vi "power_measure.vi"() -> ()   [LabVIEW 2020]
uses:
  <vilib>/ptbypt/NI_PtbyPt.lvlib
panel:
  in  "save":bool
  in  "no of data point for time":i32=100
  in  "no. of  data point for power":i32=100
  out "Avg_time":dbl format="%0.2f"
  out "average_power":dbl
  out "Time (s)":dbl
  out "Date":string
  in  "Filename":string
  in  "path":path
  out "Waveform Chart":waveform(dbl)(graph)
  out "Power":dbl
  in  "stop":bool
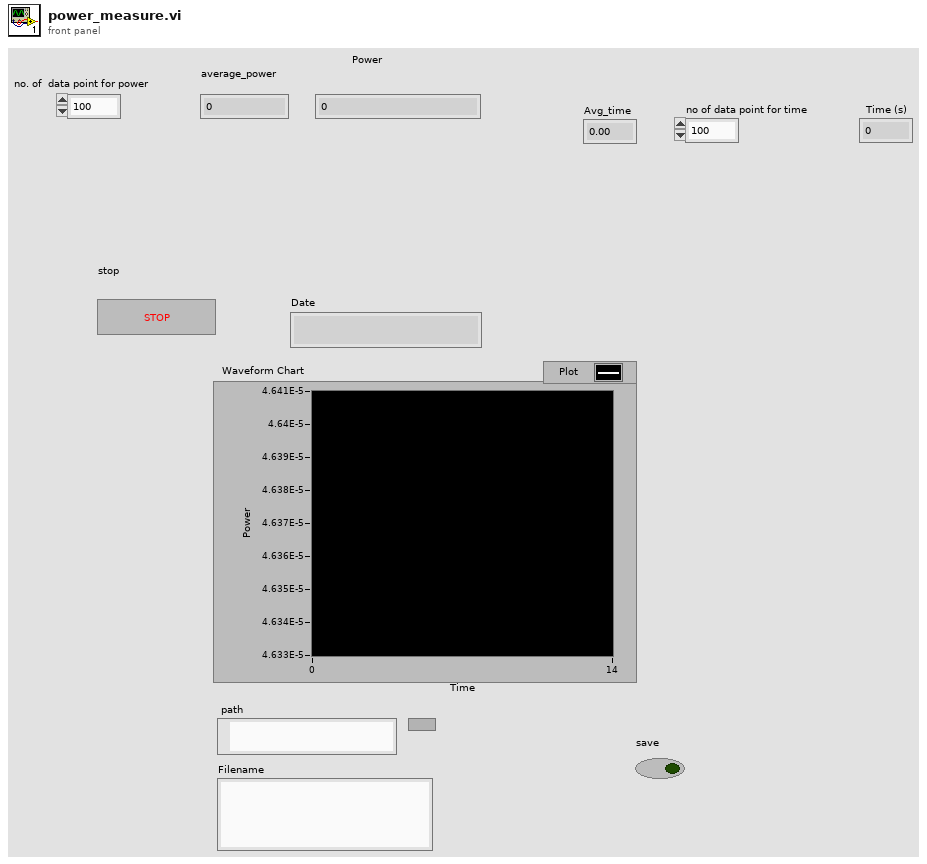
[diagram p1: front panel]
types:
  T1 = enum16{"open", "replace", "create", "open or create", "replace or create", "replace or create with confirmation"}
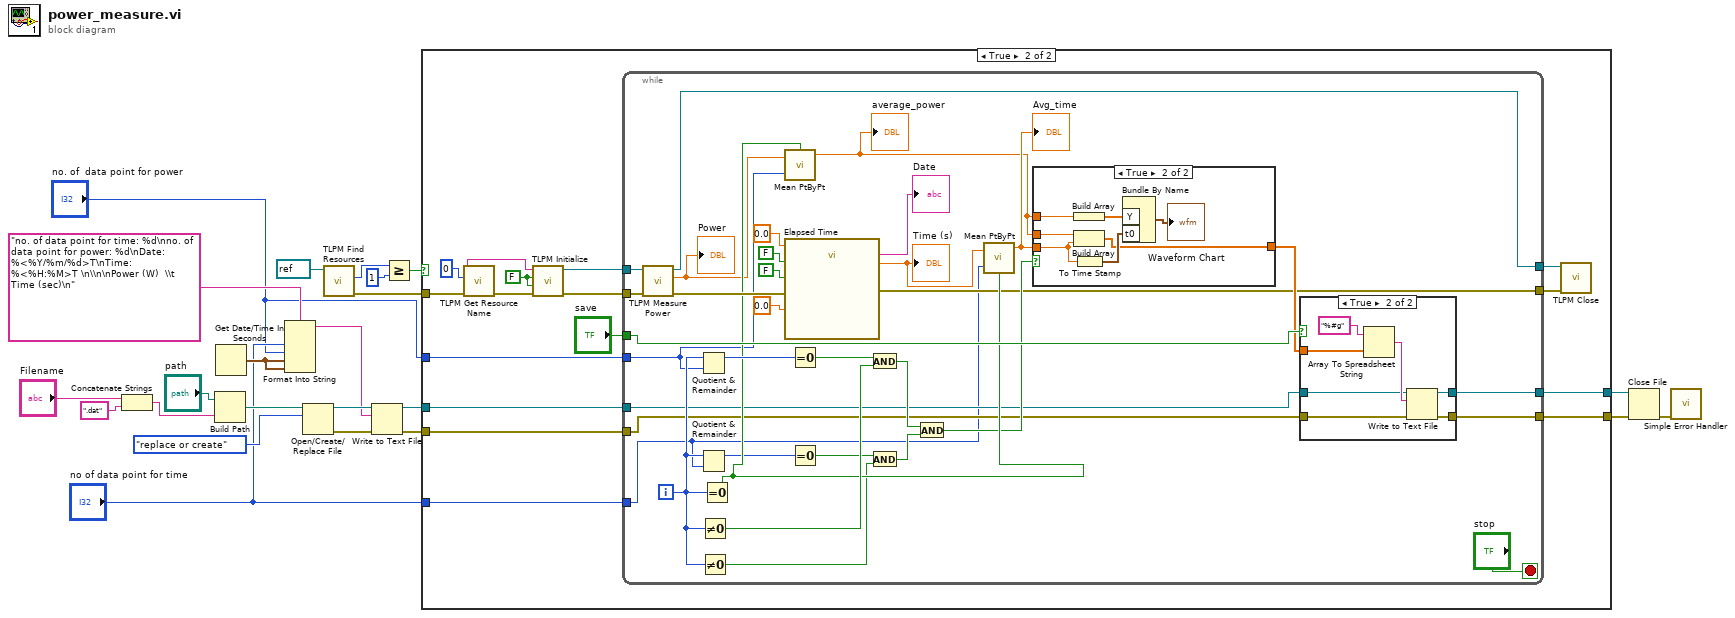
[diagram p0: block diagram]
diagram:
  n1 = Concatenate Strings("Filename", ".dat" ("string")) -> (w17:string)
  n2 = Build Path(base path="path", name or relative path=w17) -> (appended path=w14:path)
  n3 = Get Date/Time In Seconds() -> (seconds since 1Jan1904=w5:timestamp)
  n4 = Format Into String(format string="no. of data point for time: %d\nno. of data point for power: %d\nDate: %<%Y/%m/%d>T\nTime: %<%H:%M>T \n\\n\nPower (W)  \\t  Time (sec)\n", "no of data point for time", "no. of  data point for power", w5, w5) -> (resulting string=w3:string)  [unwired: 2 in, 1 out]
  n5 = Open/Create/Replace File(file path (use dialog)=w14, operation (0:open)=T1."replace or create") -> (refnum out=w12:refnum<file>, error out=w11:errorcluster)  [unwired: 4 in, 1 out]
  n6 = call <instrlib>:"TLPM Find Resources.vi"("instrument handle"=refnum<visa-resource-name> refnum) -> ("error out"=w15:errorcluster, "Resource Count"=w21:u32)  [unwired: 8 in, 1 out]
  n7 = Write to Text File(file (use dialog)=w12, text=w3, error in=w11) -> (refnum out=w10:refnum<file>, error out=w8:errorcluster)  [unwired: 1 in, 1 out]
  n8 = Greater Or Equal?(x=w21, y=u32 1) -> (x >= y?=w22:bool)
  n9 = case shown="True" w22 {
    tunnel: w15 -> [_ w34]
    tunnel: w10 -> [w24 w32]
    tunnel: [w24 w31] -> w9
    tunnel: w8 -> [w25 w30]
    tunnel: [w25 w29] -> w7
    tunnel: "no. of  data point for power" -> [_ w28]
    tunnel: "no of data point for time" -> [_ w27]
    frame False {
    }
    frame True {
      w37 = FALSE ("ID Query (Do Query)")
      n10 = call <instrlib>:"TLPM Get Resource Name.vi"("error in (no error)"=w34, "Index (0)"=u32 0) -> ("error out"=w35:errorcluster, "Resource Name"=w40:string)  [unwired: 7 in, 1 out]
      n11 = call <instrlib>:"TLPM Initialize.vi"("error in (no error)"=w35, "Reset Device (Reset Device)"=w37, "ID Query (Do Query)"=w37, "resource name"=w40) -> ("error out"=w36:errorcluster, "instrument handle out"=w39:refnum<visa-resource-name>)  [unwired: 6 in]
      n12 = while {
        tunnel: w39 -> [w74]
        tunnel: [w73] -> w38
        tunnel: "save" -> [w71]
        tunnel: w36 -> [w72]
        tunnel: [w50] -> w33
        tunnel: w32 -> [w49]
        tunnel: [w48] -> w31
        tunnel: w30 -> [w47]
        tunnel: [w46] -> w29
        tunnel: w28 -> [w45]
        tunnel: w27 -> [w42]
        i -> [w58]
        stop <- "stop" stop-if-true
        n13 = call <instrlib>:"TLPM Measure Power.vi"("error in (no error)"=w72, "instrument handle"=w74) -> ("error out"=w70:errorcluster, "Power"=w44:dbl, "instrument handle out"=w73:refnum<visa-resource-name>)  [unwired: 7 in]
        "Power" <- w44
        n14 = Quotient & Remainder(x=w58, y=w45) -> (x-y*floor(x/y)=w64:i32)  [unwired: 1 out]
        n15 = Quotient & Remainder(x=w58, y=w42) -> (x-y*floor(x/y)=w59:i32)  [unwired: 1 out]
        n16 = Not Equal To 0?(x=w58) -> (x != 0?=w62:bool)
        n17 = Not Equal To 0?(x=w58) -> (x != 0?=w56:bool)
        n18 = Equal To 0?(x=w58) -> (x = 0?=w61:bool)
        n19 = call <vilib>:"Mean PtByPt.vi"("x"=w44, "sample length"=w45, "initialize"=w61) -> ("mean"=w52:dbl)  [unwired: 1 in, 1 out]
        "average_power" <- w52
        n20 = call "Elapsed Time"("Time Target (s)"=0.0, "Reset"=FALSE ("Auto Reset"), "Auto Reset"=FALSE ("Reset"), "error in (no error)"=w70, "Set Start Time (s)"=0.0) -> ("Present Text"=→"Date":string, "Elapsed Time (s)"=w43:dbl, "error out"=w50:errorcluster)  [unwired: 7 in, 5 out]
        "Time (s)" <- w43
        n21 = Equal To 0?(x=w64) -> (x = 0?=w63:bool)
        n22 = Equal To 0?(x=w59) -> (x = 0?=w57:bool)
        n23 = And(x=w63, y=w62) -> (x .and. y?=w54:bool)
        n24 = And(x=w57, y=w56) -> (x .and. y?=w55:bool)
        n25 = And(x=w54, y=w55) -> (x .and. y?=w53:bool)
        n26 = call <vilib>:"Mean PtByPt.vi"("x"=w43, "sample length"=w42, "initialize"=w61) -> ("mean"=w60:dbl)  [unwired: 1 in, 1 out]
        "Avg_time" <- w60
        n27 = case shown="True" w53 {
          tunnel: w52 -> [_ w81]
          tunnel: w60 -> [_ w78]
          tunnel: w52 -> [_ w77]
          tunnel: [_ w76] -> w51
          frame False {
          }
          frame True {
            n28 = Build Array(w81) -> (w80:dbl[])
            n29 = Build Array(w77, w78) -> (w76:dbl[])
            n30 = To Time Stamp(1:w78) -> (0:w79:timestamp)
            n31 = Bundle By Name("Y"=w80, "t0"=w79) -> (→"Waveform Chart":waveform(dbl))  [unwired: 1 in]
          }
        }
        n32 = case shown="True" w71 {
          tunnel: w51 -> [_ w89]
          tunnel: w49 -> [w83 w88]
          tunnel: [w83 w87] -> w48
          tunnel: w47 -> [w84 w86]
          tunnel: [w84 w85] -> w46
          frame False {
          }
          frame True {
            n33 = Array To Spreadsheet String(array=w89, 3:"%#g" ("format string")) -> (spreadsheet string=w91:string)  [unwired: 1 in]
            n34 = Write to Text File(file (use dialog)=w88, text=w91, error in=w86) -> (refnum out=w87:refnum<file>, error out=w85:errorcluster)  [unwired: 1 in, 1 out]
          }
        }
      }
      n35 = call <instrlib>:"TLPM Close.vi"("error in (no error)"=w33, "instrument handle"=w38) -> ()  [unwired: 9 in, 1 out]
    }
  }
  n36 = Close File(refnum=w9, error in=w7) -> (error out=w6:errorcluster)  [unwired: 1 out]
  n37 = call <vilib>:"Simple Error Handler.vi"("error in (no error)"=w6) -> ()  [unwired: 1 in, 8 out]
